vi "Run 1.vi"   [LabVIEW 2016]
types:
  T1 = typedef "LVHSConnector.ctl" = refnum<class "BrickReference.lvclass">
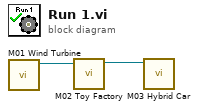
[diagram p0: block diagram]
diagram:
  n1 = call "M01 Wind Turbine.vi"() -> ("EV3 out"=w2:T1)  [unwired: 11 in]
  n2 = call "M02 Toy Factory.vi"("EV3 in"=w2) -> ("NXT/EV3"=w1:T1)  [unwired: 10 in]
  n3 = call "M03 Hybrid Car.vi"("EV3 in"=w1) -> ()  [unwired: 10 in, 1 out]
